vi "ReadFileForCurrentList.vi"(8 "error in":errorcluster, 11 "CurrentList file path":path) -> (0 "error out":errorcluster, 3 "CurrentList out":string[][](array[string]))   [LabVIEW 2020]
panel:
  in  "Waveform List":string[][](table)=[["1", ".01"], ["2", ".01"], ["3", ".01"], ["4\n", ".01"], ["3", ".01"], ["2", ".01"], ["1", ".01"], ["0", ".01"]]
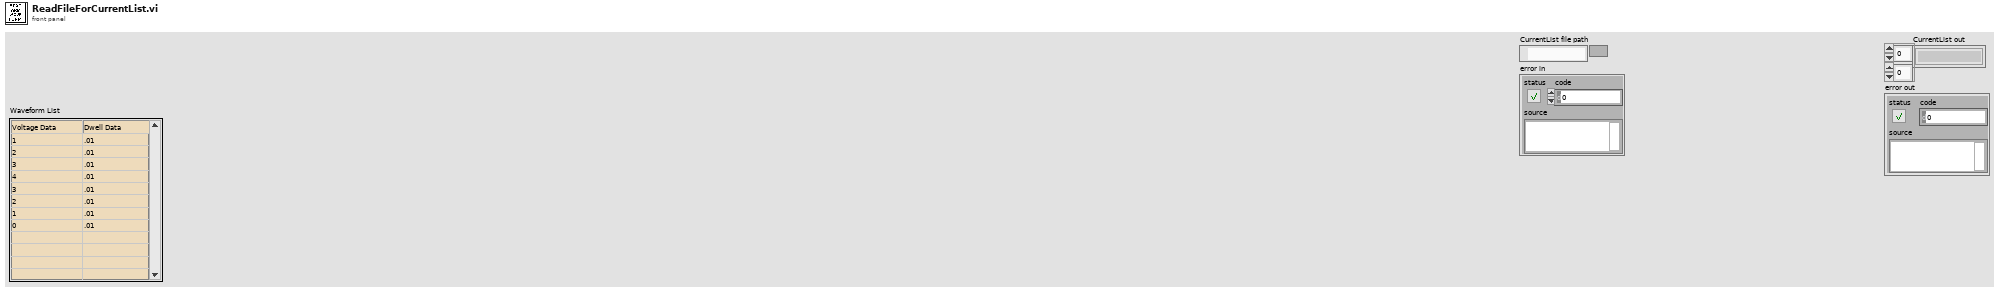
[diagram p1: front panel]
types:
  T1 = enum16{"open", "replace", "create", "open or create", "replace or create", "replace or create with confirmation"}
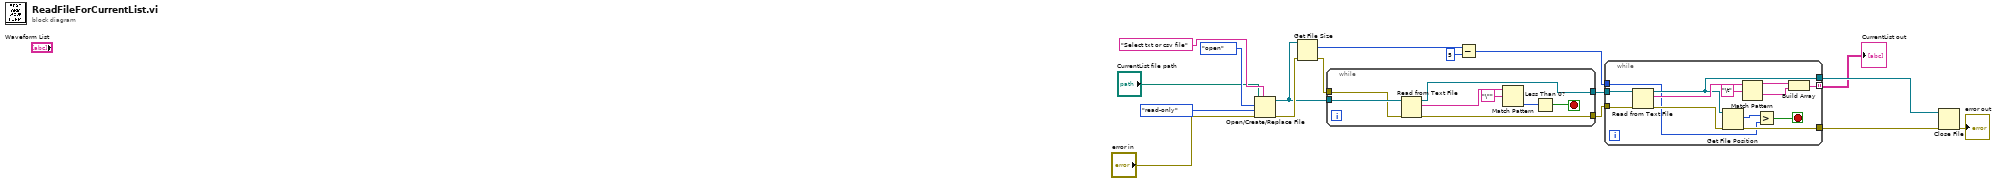
[diagram p0: block diagram]
diagram:
  n1 = Open/Create/Replace File(file path (use dialog)="CurrentList file path", error in="error in", prompt="Select txt or csv file", operation (0:open)=T1."open", access (0:read/write)=enum16{"read/write", "read-only", "write-only"}."read-only") -> (refnum out=w12:refnum<file>, error out=w13:errorcluster)  [unwired: 1 in, 1 out]
  n2 = Get File Size(file=w12, error in=w13) -> (size (in bytes)=w7:i64, 0:w8:errorcluster)  [unwired: 1 out]
  n3 = while {
    tunnel: w12 -> [w25]
    tunnel: [w24] -> w11
    tunnel: [w19] -> w9
    tunnel: w8 -> [w18]
    stop <- w20 stop-if-true
    n4 = Read from Text File(file (use dialog)=w25, error in=w18) -> (refnum out=w24:refnum<file>, text=w23:string, error out=w19:errorcluster)  [unwired: 2 in, 1 out]
    n5 = Match Pattern(string=w23, regular expression="\"") -> (offset past match=w21:i32)  [unwired: 1 in, 3 out]
    n6 = Less Than 0?(x=w21) -> (x < 0?=w20:bool)
  }
  n7 = Subtract(x=w7, y=i64 5) -> (x-y=w5:i64)
  n8 = while {
    tunnel: w11 -> [w38]
    tunnel: [w33] -> w14
    tunnel: [w31] -> w10
    tunnel: w9 -> [w30]
    tunnel: w5 -> [w29]
    tunnel: [w26] -> w4 mode=indexing
    stop <- w35 stop-if-true
    n9 = Read from Text File(file (use dialog)=w38, error in=w30) -> (refnum out=w33:refnum<file>, text=w37:string, error out=w32:errorcluster)  [unwired: 2 in, 1 out]
    n10 = Get File Position(4:w32, 7:w33) -> (0:w31:errorcluster, 2:w34:i64)  [unwired: 1 out]
    n11 = Match Pattern(string=w37, regular expression="\t") -> (before substring=w28:string, after substring=w27:string)  [unwired: 1 in, 2 out]
    n12 = Greater?(x=w34, y=w29) -> (0:w35:bool)
    n13 = Build Array(w28, w27) -> (w26:string[])
  }
  "CurrentList out" <- w4
  n14 = Close File(refnum=w14, error in=w10) -> (error out=→"error out":errorcluster)  [unwired: 1 out]
